vi "SMBUS Read Word Protocol.vi"(6 "WithPEC":u8, 7 "CommandCode":u8, 9 "SlaveAddr":i16, 10 "IICIndex":i32, 11 "DevIndex":i32) -> (2 "function return":i32, 3 "pData":u16[](array[numeric]))   [LabVIEW 2010, in "usb2iic.lvlib"]
doc: "int WINAPI SMBUS_ReadWordProtocol(int DevIndex,int IICIndex,short SlaveAddr,unsigned char CommandCode, unsigned short *pData,unsigned char WithPEC);"
uses:
  usb2iic.lvlib
  USB2XXX.dll
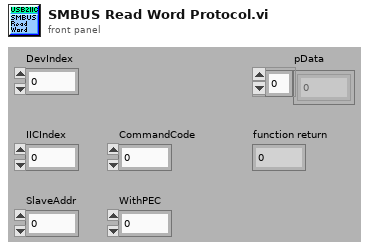
[diagram p1: front panel]
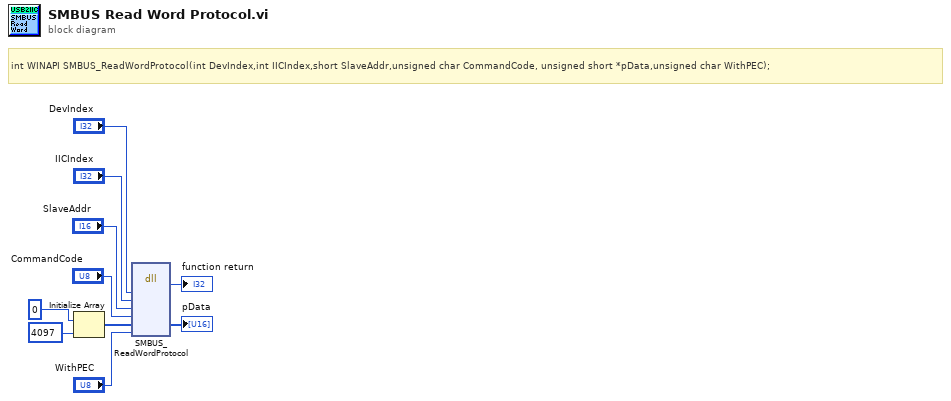
[diagram p0: block diagram]
diagram:
  # "int WINAPI SMBUS_ReadWordProtocol(int DevIndex,int IICIndex,short SlaveAddr,unsigned char CommandCode, unsigned short *pData,unsigned char WithPEC);"
  n1 = Initialize Array(u16 0 ("element"), 4097 ("dimension size")) -> (w5:u16[])
  n2 = dll-call lib="G:/OtherWork/USB2XXX_Example/trunk/Labview/PublicFiles/usb2iic/USB2XXX.*" fn="SMBUS_ReadWordProtocol"("DevIndex"="DevIndex", "IICIndex"="IICIndex", "SlaveAddr"="SlaveAddr", "CommandCode"="CommandCode", "pData"=w5, "WithPEC"="WithPEC") -> (→"function return":i32, "pData"=→"pData":u16[])  [unwired: 8 in, 2 out]
